vi "ITC503_Check_Queue.vi"(7 "error in (no error)":errorcluster, 10 "queue":refnum<queue>) -> (0 "error out":errorcluster, 1 "ITC503-Control":T1={"Setpoint (K)"=0.0, "Rate (K/min)"=3.4572, "Go to Set"=FALSE, "Set Heater SP"=FALSE, "Set NV SP"=FALSE, "Change Heater Status"=FALSE, "Change NV Status"=FALSE, "Set Auto PID"=FALSE, "Stopp"=FALSE, "Control Channel"=FALSE, "Heater SP"=0.0, "NV Setpoint"=0.0} {"Rate (K/min)" format="%#4_5f"; "Setpoint (K)" format="%6_5f"}, 3 "New Entries?":bool)   [LabVIEW 2019]
uses:
  ITC503/ITC503_control.ctl
panel:
  out "Numeric":i32
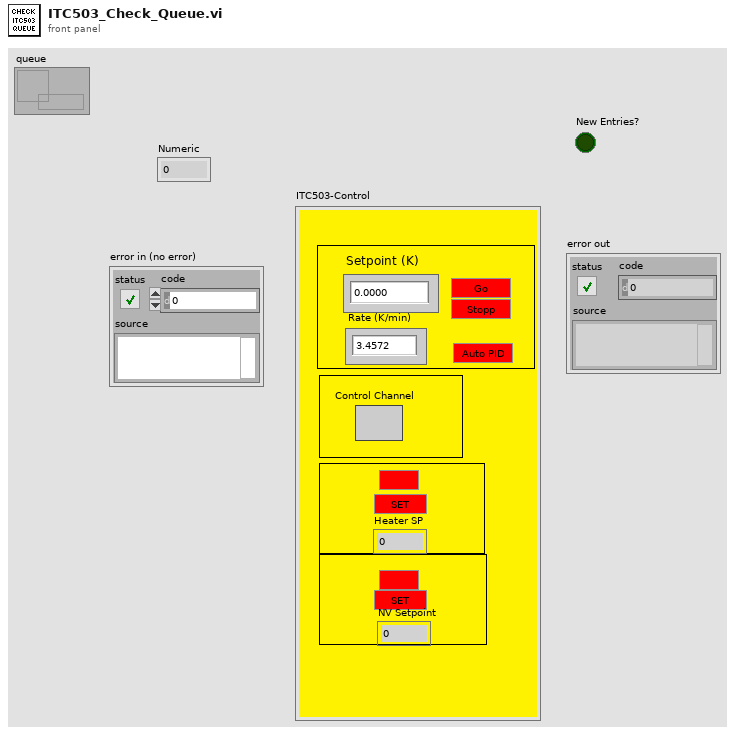
[diagram p1: front panel]
types:
  T1 = typedef "ITC503_control.ctl" = cluster{"Setpoint (K)":dbl, "Rate (K/min)":dbl, "Go to Set":bool, "Set Heater SP":bool, "Set NV SP":bool, "Change Heater Status":bool, "Change NV Status":bool, "Set Auto PID":bool, "Stopp":bool, "Control Channel":bool, "Heater SP":dbl, "NV Setpoint":dbl}
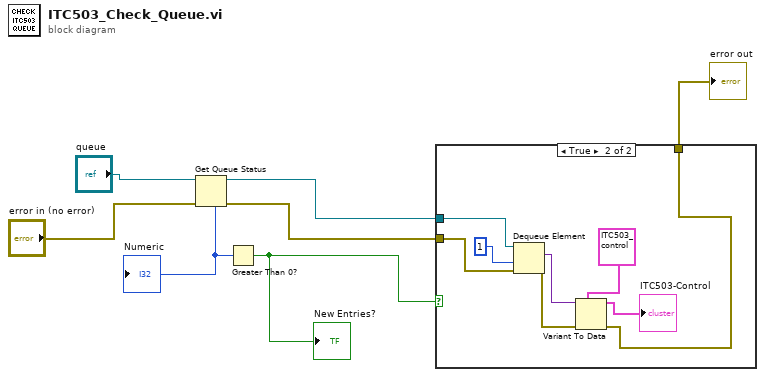
[diagram p0: block diagram]
diagram:
  n1 = Get Queue Status(queue="queue", error in (no error)="error in (no error)") -> (queue out=w4:refnum<queue>, error out=w6:errorcluster, # elements in queue=w2:i32)  [unwired: 1 in, 5 out]
  "Numeric" <- w2
  n2 = Greater Than 0?(x=w2) -> (x > 0?=w1:bool)
  "New Entries?" <- w1
  n3 = case shown="True" w1 {
    tunnel: w4 -> [_ w15]
    tunnel: w6 -> [w8 w14]
    tunnel: [w8 w9] -> w5
    frame False {
    }
    frame True {
      n4 = Dequeue Element(queue=w15, timeout in ms (-1)=1, error in (no error)=w14) -> (element=w13:variant, error out=w12:errorcluster)  [unwired: 2 out]
      n5 = Variant To Data(error in=w12, type=T1 {"Setpoint (K)"=0.0, "Rate (K/min)"=3.4572, "Go to Set"=FALSE, "Set Heater SP"=FALSE, "Set NV SP"=FALSE, "Change Heater Status"=FALSE, "Change NV Status"=FALSE, "Set Auto PID"=FALSE, "Stopp"=FALSE, "Control Channel"=FALSE, "Heater SP"=0.0, "NV Setpoint"=0.0} ("ITC503-Control"), Variant=w13) -> (data=→"ITC503-Control":T1, error out=w9:errorcluster)
    }
  }
  "error out" <- w5
